vi "oldVers.vi"() -> ()   [LabVIEW 2021]
uses:
  <vilib>/myRIO/Common/Instrument Driver Framework/myRIO v1.0/Encoder/typedefs/Encoder Signal Mode.ctl
  <vilib>/Platform/TimedLoop/XDataNode/timing_clust.ctl
  <vilib>/Platform/TimedLoop/XDataNode/nitl_modes.ctl
  <vilib>/Platform/TimedLoop/XDataNode/wakeup.ctl
  <vilib>/myRIO/Common/Instrument Driver Framework/myRIO v1.0/UART/vis/myRIO v1.0 Close UART.vi
  <vilib>/Utility/error.llb/Error Cluster From Error Code.vi
  <vilib>/myRIO/Common/Instrument Driver Framework/myRIO v1.0/Encoder/vis/myRIO v1.0 Read Encoder.vi
  <vilib>/myRIO/Common/Instrument Driver Framework/myRIO v1.0/DIO/vis/myRIO v1.0 Read DIO.vi
  <vilib>/myRIO/Common/Instrument Driver Framework/myRIO v1.0/PWM/vis/myRIO v1.0 Write PWM.vi
  <vilib>/myRIO/Common/Instrument Driver Framework/Utilities/vis/FPGA Ref Manager.vi
  <vilib>/myRIO/Common/Instrument Driver Framework/myRIO v1.0/myRIO v1.0 Reset FPGA.vi
  <vilib>/myRIO/Common/Instrument Driver Framework/myRIO v1.0/IRQ/vis/myRIO v1.0 IRQ Info FGV.vi
  <vilib>/myRIO/Common/Instrument Driver Framework/myRIO v1.0/IRQ/vis/myRIO v1.0 Timer IRQ Info FGV.vi
  <vilib>/myRIO/Common/Instrument Driver Framework/myRIO v1.0/IRQ/vis/myRIO v1.0 ISR Agent.vi
  <vilib>/myRIO/Instrument Drivers/Utilities/vis/Reset Index.vi
  <vilib>/myRIO/Common/Instrument Driver Framework/myRIO v1.0/Resource Manager/vis/myRIO v1.0 Block Write Resource Manager.vi
  <vilib>/Platform/TimedLoop/XDataNode/XDataNode.xnode
  <vilib>/myRIO/Instrument Drivers/Onboard IO/Encoder/Encoder.lvlib
  <vilib>/myRIO/Instrument Drivers/Onboard IO/PWM/PWM.lvlib
  <vilib>/myRIO/Instrument Drivers/Utilities/Utilities.lvlib
  <vilib>/Platform/TimedLoop/XDataNode/XDNodeRunTimeDep.lvlib
  <vilib>/myRIO/Instrument Drivers/Onboard IO/DIO/DIO.lvlib
panel:
  out "diff":dbl
  in  "LS":bool
  out "+pwm":dbl
  out "-pwm":dbl
  out "Last Measure":dbl
  in  "stop":bool
  in  "Measure":bool
  in  "X":dbl(slide) scale=-20.0..50.0
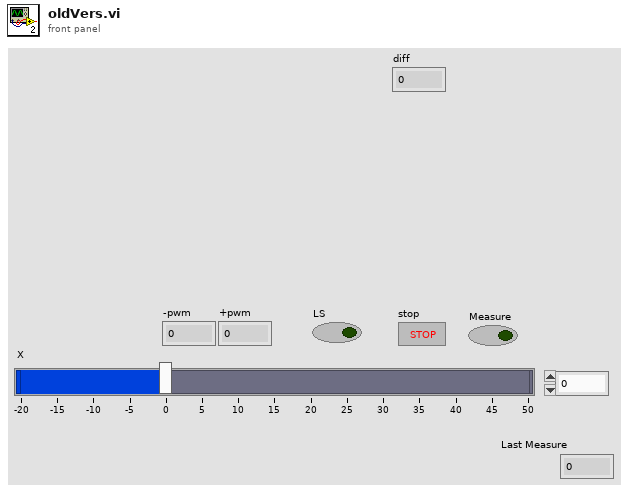
[diagram p1: front panel]
types:
  T1 = typedef "XDNodeRunTimeDep.lvlib/timing_clust.ctl" = cluster{"Expected End [f-1]":u64, "Actual End [f-1]":u64, "Finished Late? [f-1]":bool, "Expected End [i-1]":u64, "Actual End [i-1]":u64, "Finished Late? [i-1]":bool, "Expected Start [i]":u64, "Actual Start [i]":u64, "Expected Start [f]":u64, "Actual Start [f]":u64, "Source Name":string, "Structure Name":string, "Period":i64, "Deadline":i64, "Offset":i64, "Start":i64, "Priority":i32, "Timeout":i32, "Mode":T2, "Wakeup Reason":T3, "Error":errorcluster, "Source Type":string, "Secondary Source Type":string, "Global End Time":u64, "Global Start Time":u64, "Frame Duration":u64, "Iteration Duration":u64, "Assigned CPU":i32, "I/O Scan Engine Mode":u32}
  T2 = typedef "XDNodeRunTimeDep.lvlib/nitl_modes.ctl" = enum32{"No Change", "Process missed periods, maintain original phase", "Discard missed periods, maintain original phase", "Process missed periods, ignore original phase", "Discard missed periods, ignore original phase"}
  T3 = typedef "XDNodeRunTimeDep.lvlib/wakeup.ctl" = enum32{"Normal", "Aborted", "Asynchronous wakeup", "Timing source error", "Timed loop error", "Timeout"}
  T4 = enum8{"Enabled", "Disabled", "Disabled and Grayed Out"}
  T5 = typedef "Encoder Signal Mode.ctl" = enum16{"Quadrature phase signal", "Step and direction signal"}
  T6 = typedef "Encoder.lvlib/Encoder Reference.ctl" = cluster{"myRIO Reference":T7, "Encoder Channels Enum":T11}
  T7 = typedef "myRIO Generic Hardware Reference.ctl" = cluster{"myRIO Model":T8, "myRIO Hardware Reference":T9}
  T8 = typedef "Hardware Version Enum.ctl" = enum16{"Unknown", "myRIO-1900", "myRIO-1950", "roboRIO", "NI ELVIS RIO CM", "ELVIS III"}
  T9 = typedef "myRIO v1.0 Reference.ctl" = cluster{"Generic FPGA Reference":T10, "Allow multiple opens":bool}
  T10 = typedef "Generic FPGA Reference.ctl" = refnum<k20>
  T11 = typedef "Encoder Channels Enum.ctl" = enum16{"Not Connected", "C/ENC0", "C/ENC1", "A/ENC", "A/ENC0", "A/ENC1", "A/ENC2", "A/ENC3", "A/ENC4", "A/ENC5", "A/ENC6", "A/ENC7", "A/ENC8", "A/ENC9", "B/ENC", "B/ENC0", "B/ENC1", "B/ENC2", "B/ENC3", "B/ENC4", "B/ENC5", "B/ENC6", "B/ENC7", "B/ENC8", "B/ENC9", "DIO/ENC0", "DIO/ENC1", "DIO/ENC2", "DIO/ENC3", "DIO/ENC4"}
  T12 = typedef "DIO.lvlib/DIO Reference.ctl" = cluster{"myRIO Reference":T7, "DIO Channels List":T13}
  T13 = typedef "DIO Channels List.ctl" = T14[]
  T14 = typedef "DIO Channels Enum.ctl" = enum16{"Not Connected", "C/DIO0", "C/DIO1", "C/DIO2", "C/DIO3", "C/DIO4", "C/DIO5", "C/DIO6", "C/DIO7", "A/DIO0", "A/DIO1", "A/DIO2", "A/DIO3", "A/DIO4", "A/DIO5", "A/DIO6", "A/DIO7", "A/DIO8", "A/DIO9", "A/DIO10", "A/DIO11", "A/DIO12", "A/DIO13", "A/DIO14", "A/DIO15", "A/DIO16", "A/DIO17", "A/DIO18", "A/DIO19", "B/DIO0", "B/DIO1", "B/DIO2", "B/DIO3", "B/DIO4", "B/DIO5", "B/DIO6", "B/DIO7", "B/DIO8", "B/DIO9", "B/DIO10", "B/DIO11", "B/DIO12", "B/DIO13", "B/DIO14", "B/DIO15", "B/DIO16", "B/DIO17", "B/DIO18", "B/DIO19", "LED0", "LED1", "LED2", "LED3", "Button0", "DIO/DIO0", "DIO/DIO1", "DIO/DIO2", "DIO/DIO3", "DIO/DIO4", "DIO/DIO5", "DIO/DIO6", "DIO/DIO7", "DIO/DIO8", "DIO/DIO9", "SPI/CS0", "SPI/CS1", "SPI/CS2", "SPI/CS3", "LED RADIO (Green)", "LED RADIO (Red)", "LED COMM (Green)", "LED COMM (Red)", "LED MODE (Green)", "LED MODE (Red)"}
  T15 = typedef "PWM.lvlib/PWM Reference.ctl" = cluster{"myRIO Reference":T7, "PWM Channels Enum":T16, "PWM Configuration":T17}
  T16 = typedef "PWM Channels Enum.ctl" = enum16{"Not Connected", "C/PWM0", "C/PWM1", "A/PWM0", "A/PWM1", "A/PWM2", "A/PWM3", "A/PWM4", "A/PWM5", "A/PWM6", "A/PWM7", "A/PWM8", "A/PWM9", "A/PWM10", "A/PWM11", "A/PWM12", "A/PWM13", "A/PWM14", "A/PWM15", "A/PWM16", "A/PWM17", "A/PWM18", "A/PWM19", "B/PWM0", "B/PWM1", "B/PWM2", "B/PWM3", "B/PWM4", "B/PWM5", "B/PWM6", "B/PWM7", "B/PWM8", "B/PWM9", "B/PWM10", "B/PWM11", "B/PWM12", "B/PWM13", "B/PWM14", "B/PWM15", "B/PWM16", "B/PWM17", "B/PWM18", "B/PWM19", "PWM/PWM0", "PWM/PWM1", "PWM/PWM2", "PWM/PWM3", "PWM/PWM4", "PWM/PWM5", "PWM/PWM6", "PWM/PWM7", "PWM/PWM8", "PWM/PWM9"}
  T17 = typedef "PWM.lvlib/PWM Configuration.ctl" = cluster{"Frequency":dbl, "Duty Cycle":dbl}
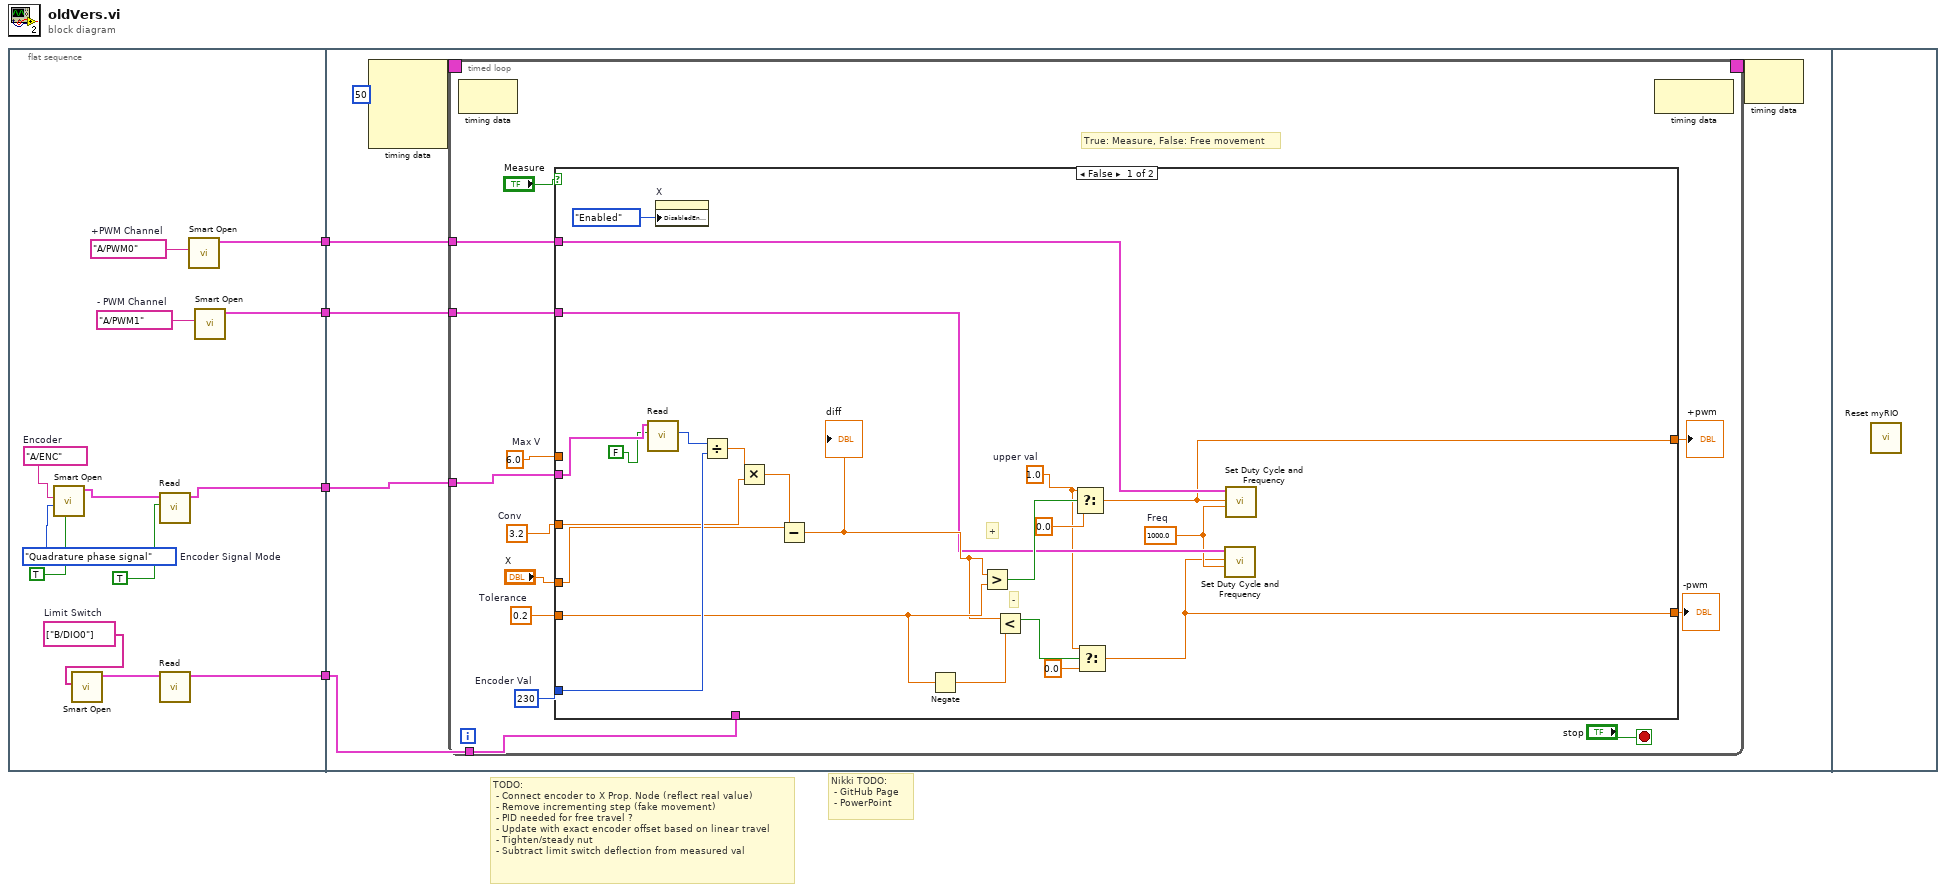
[diagram p0: block diagram]
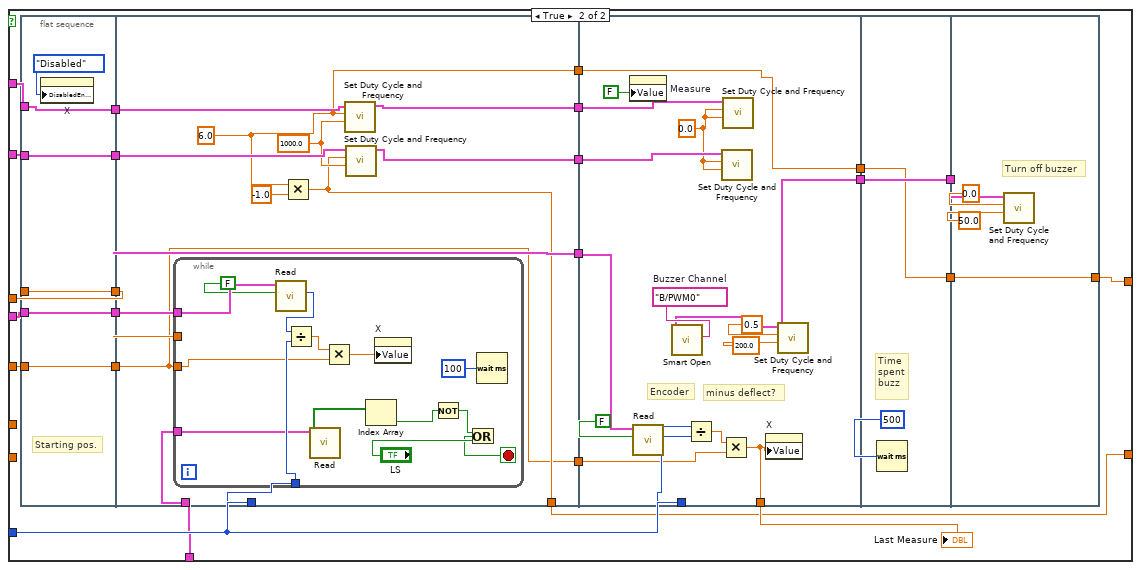
[diagram p2: hidden frame]
diagram:
  # "Nikki TODO:\n - GitHub Page \n - PowerPoint"
  # "TODO: \n - Connect encoder to X Prop. Node (reflect real value)\n - Remove incrementing step (fake movement)\n - PID needed for free travel ? \n - Update with exact encoder offset based on linear travel\n - Tighten/steady nut  \n - Subtract limit switch deflection from measured val"
  n1 = flat-sequence {
    tunnel: [w12] -> w4
    tunnel: [w9] -> w3
    tunnel: [w6] -> w2
    tunnel: [w5] -> w1
    tunnel: w4 -> [w21]
    tunnel: w3 -> [w20]
    tunnel: w2 -> [w19]
    tunnel: w1 -> [w18]
    frame #0 {
      w7 = tag "A/PWM1"  # - PWM Channel
      w8 = tag "A/PWM0"  # +PWM Channel
      w11 = tag[] ["B/DIO0"]  # Limit Switch
      w16 = Encoder_Signal_Mode."Quadrature phase signal"  # Encoder Signal Mode
      w17 = tag "A/ENC"  # Encoder
      n2 = call <vilib>:"Smart Open.vi"("Start Counter"=TRUE, "Encoder Signal Mode"=w16, "Channel Name"=w17) -> ("Encoder Ref Out"=w13:T6)  [unwired: 7 in, 1 out]
      n3 = call <vilib>:"Smart Open.vi"("Channel Names"=w11) -> ("DIO Ref Out"=w10:T12)  [unwired: 9 in, 1 out]
      n4 = call <vilib>:"Read.vi"("Reset Counter"=TRUE, "Encoder Ref In"=w13) -> ("Encoder Ref Out"=w12:T6)  [unwired: 5 in, 4 out]
      n5 = call <vilib>:"Read.vi"("DIO Ref In"=w10) -> ("DIO Ref Out"=w9:T12)  [unwired: 8 in, 2 out]
      n6 = call <vilib>:"Smart Open.vi"("Channel Name"=w8) -> ("PWM Ref Out"=w6:T15)  [unwired: 9 in, 1 out]
      n7 = call <vilib>:"Smart Open.vi"("Channel Name"=w7) -> ("PWM Ref Out"=w5:T15)  [unwired: 9 in, 1 out]
    }
    frame #1 {
      n8 = node-c288(i64 50 ("Period")) -> (w24:T1)  [unwired: 3 in]
      n9 = timed-loop {
        timing: w24 -> [_]
        timing-out: [_] -> w23
        tunnel: w21 -> [w32]
        tunnel: w20 -> [w31]
        tunnel: w19 -> [w30]
        tunnel: w18 -> [w29]
        stop <- "stop" stop-if-true
        w25 = 0.2  # Tolerance
        w26 = 3.2  # Conv
        w33 = 230  # Encoder Val
        w34 = 6.0  # Max V
        # "True: Measure, False: Free movement"
        n10 = node-c288() -> ()  [unwired: 1 in, 1 out]
        n11 = case shown="False" "Measure" {
          tunnel: "X" -> [w59 _]
          tunnel: w34 -> [_ w85]
          tunnel: w33 -> [w60 w83]
          tunnel: w32 -> [w58 w79]
          tunnel: w31 -> [_ w78]
          tunnel: w30 -> [w47 w76]
          tunnel: w29 -> [w46 w74]
          tunnel: [w41 w66] -> w28
          tunnel: [w40 w65] -> w27
          tunnel: w26 -> [w53 w64]
          tunnel: w25 -> [w51 _]
          frame False {
            w42 = 1.0  # upper val
            w44 = 1000.0  # Freq
            # "-"
            # "+"
            n12 = call <vilib>:"Read.vi"("Reset Counter"=FALSE, "Encoder Ref In"=w58) -> ("Counter Value"=w56:i32)  [unwired: 5 in, 4 out]
            n13 = property on="X" class="Slide (strict)"("DisabledEnum"=T4."Enabled" ("Disabled")) -> ()  [unwired: 2 in, 2 out]
            n14 = Divide(x=w56, y=w60) -> (x/y=w55:dbl)
            n15 = Multiply(x=w55, y=w53) -> (x*y=w54:dbl)
            n16 = Subtract(x=w59, y=w54) -> (x-y=w50:dbl)
            "diff" <- w50
            n17 = Negate(x=w51) -> (-x=w43:dbl)
            n18 = Greater?(x=w50, y=w51) -> (0:w52:bool)
            n19 = Less?(x=w50, y=w43) -> (x < y?=w49:bool)
            n20 = Select(t=w42, s=w52, f=0.0 ("t")) -> (s? t:f=w41:dbl)
            n21 = Select(t=w42, s=w49, f=0.0) -> (s? t:f=w40:dbl)
            n22 = call <vilib>:"Set Duty Cycle and Frequency.vi"("Frequency [Hz]"=w44, "Duty Cycle"=w40, "PWM Ref In"=w46) -> ()  [unwired: 6 in, 2 out]
            n23 = call <vilib>:"Set Duty Cycle and Frequency.vi"("Frequency [Hz]"=w44, "Duty Cycle"=w41, "PWM Ref In"=w47) -> ()  [unwired: 6 in, 2 out]
          }
          frame True {
            n24 = flat-sequence {
              tunnel: w85 -> [w91]
              tunnel: [w91] -> w84
              tunnel: [w89] -> w80
              tunnel: w79 -> [w89]
              tunnel: w76 -> [w88]
              tunnel: [w88] -> w75
              tunnel: w74 -> [w87]
              tunnel: [w87] -> w73
              tunnel: w64 -> [w86]
              tunnel: [w86] -> w63
              tunnel: w84 -> [w104]
              tunnel: w83 -> [w103]
              tunnel: w80 -> [w101]
              tunnel: w78 -> [w102]
              tunnel: [w101] -> w77
              tunnel: w75 -> [w100]
              tunnel: w73 -> [w99]
              tunnel: [w96] -> w72
              tunnel: [w95] -> w71
              tunnel: [w94] -> w69
              tunnel: [w93] -> w65
              tunnel: w63 -> [w92]
              tunnel: [w92] -> w62
              tunnel: w83 -> [w134]
              tunnel: [w129] -> w82
              tunnel: w77 -> [w128]
              tunnel: w72 -> [w125]
              tunnel: w71 -> [w124]
              tunnel: [w121] -> w70
              tunnel: w69 -> [w120]
              tunnel: [w120] -> w68
              tunnel: w62 -> [w119]
              tunnel: w82 -> [w137]
              tunnel: [w137] -> w81
              tunnel: w68 -> [w136]
              tunnel: [w136] -> w67
              tunnel: w81 -> [w140]
              tunnel: w67 -> [w139]
              tunnel: [w139] -> w66
              frame #0 {
                # "Starting pos."
                n25 = property on="X" class="Slide (strict)"("DisabledEnum"=T4."Disabled" ("Disabled")) -> ()  [unwired: 2 in, 2 out]
              }
              frame #1 {
                w97 = 1000.0 ("Frequency [Hz]")
                w94 = 6.0 ("Duty Cycle")
                n26 = while {
                  tunnel: w104 -> [_]
                  tunnel: w103 -> [w117]
                  tunnel: w101 -> [w115]
                  tunnel: w102 -> [w112]
                  tunnel: w92 -> [w106]
                  stop <- w110 stop-if-true
                  n27 = call <vilib>:"Read.vi"("Reset Counter"=FALSE, "Encoder Ref In"=w115) -> ("Counter Value"=w113:i32)  [unwired: 5 in, 4 out]
                  n28 = Divide(x=w113, y=w117) -> (x/y=w107:dbl)
                  n29 = call <vilib>:"Read.vi"("DIO Ref In"=w112) -> ("Values"=w111:bool[])  [unwired: 8 in, 2 out]
                  n30 = Multiply(x=w107, y=w106) -> (x*y=w105:dbl)
                  n31 = Index Array(array=w111) -> (element=w109:bool)  [unwired: 1 in]
                  n32 = property on="X" class="Slide (strict)"("Value"=w105) -> ()  [unwired: 2 in, 2 out]
                  n33 = Not(x=w109) -> (.not. x?=w108:bool)
                  n34 = Or(x=w108, y="LS") -> (x .or. y?=w110:bool)
                  n35 = Wait (ms)(milliseconds to wait=u32 100) -> ()  [unwired: 1 out]
                }
                n36 = Multiply(x=w94, y=-1.0) -> (x*y=w93:dbl)
                n37 = call <vilib>:"Set Duty Cycle and Frequency.vi"("Frequency [Hz]"=w97, "Duty Cycle"=w94, "PWM Ref In"=w100) -> ("PWM Ref Out"=w96:T15)  [unwired: 6 in, 1 out]
                n38 = call <vilib>:"Set Duty Cycle and Frequency.vi"("Frequency [Hz]"=w97, "Duty Cycle"=w93, "PWM Ref In"=w99) -> ("PWM Ref Out"=w95:T15)  [unwired: 6 in, 1 out]
              }
              frame #2 {
                w133 = tag "B/PWM0"  # Buzzer Channel
                w123 = 0.0 ("Step size (Duty)")
                # "minus deflect?"
                # "Encoder"
                n39 = property on="Measure" class="Bool (strict)"("Value"=FALSE ("State control")) -> ()  [unwired: 2 in, 2 out]
                n40 = call <vilib>:"Read.vi"("Reset Counter"=FALSE, "Encoder Ref In"=w128) -> ("Counter Value"=w126:i32)  [unwired: 5 in, 4 out]
                n41 = call <vilib>:"Smart Open.vi"("Channel Name"=w133) -> ("PWM Ref Out"=w132:T15)  [unwired: 9 in, 1 out]
                n42 = Divide(x=w126, y=w134) -> (x/y=w122:dbl)
                n43 = Multiply(x=w122, y=w119) -> (x*y=w121:dbl)
                n44 = call <vilib>:"Set Duty Cycle and Frequency.vi"("Frequency [Hz]"=w123, "Duty Cycle"=w123, "PWM Ref In"=w124) -> ()  [unwired: 6 in, 2 out]
                n45 = call <vilib>:"Set Duty Cycle and Frequency.vi"("Frequency [Hz]"=w123, "Duty Cycle"=w123, "PWM Ref In"=w125) -> ()  [unwired: 6 in, 2 out]
                n46 = property on="X" class="Slide (strict)"("Value"=w121) -> ()  [unwired: 2 in, 2 out]
                n47 = call <vilib>:"Set Duty Cycle and Frequency.vi"("Frequency [Hz]"=200.0, "Duty Cycle"=0.5, "PWM Ref In"=w132) -> ("PWM Ref Out"=w129:T15)  [unwired: 6 in, 1 out]
              }
              frame #3 {
                # "Time\nspent\nbuzz"
                n48 = Wait (ms)(milliseconds to wait=u32 500) -> ()  [unwired: 1 out]
              }
              frame #4 {
                # "Turn off buzzer"
                n49 = call <vilib>:"Set Duty Cycle and Frequency.vi"("Frequency [Hz]"=50.0 ("Freq [Hz]"), "Duty Cycle"=0.0, "PWM Ref In"=w140) -> ()  [unwired: 6 in, 2 out]
              }
            }
            "Last Measure" <- w70
          }
        }
        "+pwm" <- w28
        "-pwm" <- w27
        n50 = node-c288() -> ()  [unwired: 1 in, 1 out]
      }
      n51 = node-c288(w23) -> ()  [unwired: 1 out]
    }
    frame #2 {
      n52 = call <vilib>:"Reset myRIO.vi"() -> ()  [unwired: 11 in, 1 out]
    }
  }
